vi "物体外形识别.vi"() -> ()   [LabVIEW 2018]
panel:
  out "error out":errorcluster
  in  "Settings":T1={"Objects"=0, "Threshold"=128, "Reject Border"=FALSE, "Fill Holes"=FALSE, "Min Object Size"=FALSE, "Min Size"=3, "Max Object Size"=FALSE, "Max Size"=100, "Show Search Area"=FALSE, "Show Center"=TRUE, "Show Bounding Box"=TRUE} {"Objects" items=["Bright Objects", "Dark Objects"]; "Threshold" min=1 max=999999999 step=1; "Max Size" min=1 max=999999999 step=1; "Min Size" min=1 max=999999999 step=1}
  out "Number of Objects":i32
  in  "Image Type":T2 items=["Grayscale (U8)", "Grayscale (I16)", "Grayscale (SGL)", "Complex (CSG)", "RGB (U32)", "HSL (U32)", "RGB (U64)", "Grayscale (U16)"]
  out "Image":T3(plugin-control)
  in  "File Path":path
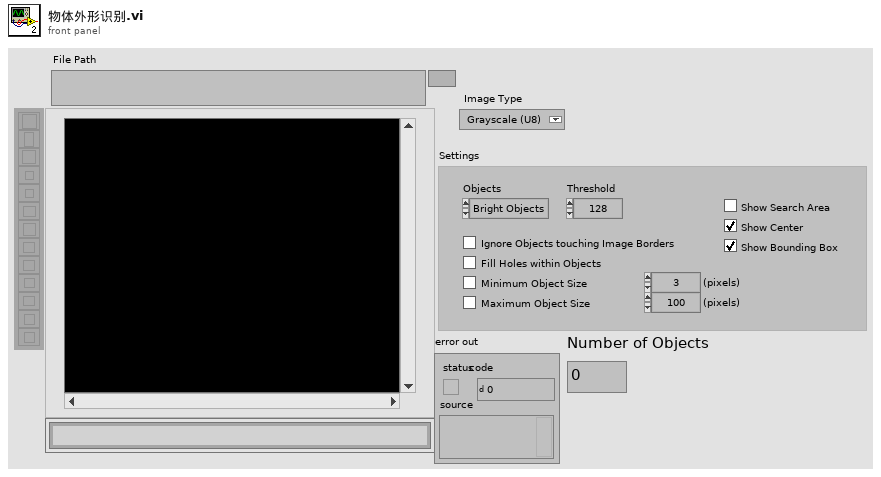
[diagram p1: front panel]
types:
  T1 = cluster{"Objects":u16, "Threshold":i32, "Reject Border":bool, "Fill Holes":bool, "Min Object Size":bool, "Min Size":i32, "Max Object Size":bool, "Max Size":i32, "Show Search Area":bool, "Show Center":bool, "Show Bounding Box":bool}
  T2 = typedef "Image Type" = u32
  T3 = typedef "IMAQ Image.ctl" = refnum<image>
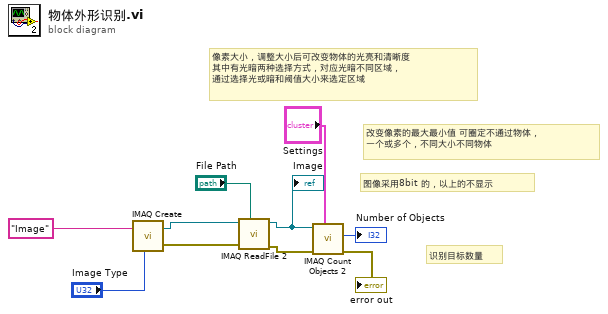
[diagram p0: block diagram]
diagram:
  # "图像采用8bit 的，以上的不显示"
  # "改变像素的最大最小值 可圈定不通过物体，\n一个或多个，不同大小不同物体"
  # "识别目标数量"
  # "像素大小，调整大小后可改变物体的光亮和清晰度\n其中有光暗两种选择方式，对应光暗不同区域，\n通过选择光或暗和阈值大小来选定区域"
  n1 = call "IMAQ Create"("Image Name"="Image", "Image Type"="Image Type") -> ("New Image"=w10:T3, "error out"=w9:errorcluster)  [unwired: 3 in]
  n2 = call "IMAQ ReadFile 2"("File Path"="File Path", "error in (no error)"=w9, "Image"=w10) -> ("error out"=w8:errorcluster, "Image Out"=w4:T3)  [unwired: 4 in, 3 out]
  "Image" <- w4
  n3 = call "IMAQ Count Objects 2"("Settings"="Settings", "error in (no error)"=w8, "Image"=w4) -> ("error out"=→"error out":errorcluster, "Number of Objects"=→"Number of Objects":i32)  [unwired: 4 in, 3 out]
